vi "pp3_updateSideState.vi"(8 "error in (no error)":errorcluster, 9 "log queue in":refnum<queue>, 10 "Daq config In":T1={"Sound AO"="Dev6/ao0", "Shock intesity AO"="Dev6/ao1", "Code_LED DO"="Dev6/port1:2", "Switch DI"="Dev6/port1/line0", "Webcam"="cam9", "Sound AO task"="", "Sound card task"=0, "Shock intensity AO task"="", "Code_LED DO task"="", "Switch DI task"="", "AO <=> Sound card"=FALSE, "Sound card"=0, "sample rate"=100000.0, "Variable shock"=TRUE, "Webcam on"=FALSE, "Waveform memo"={"t0"=timestamp(0 s since 1904-01-01), "dt"=1.0, "Y"=[]}, "Tone trigger"="PFI1", "Master-9 DO"="", "Master-9 DO task"="Dev6/port0/line5:7"} {"sample rate" min=8000.0; "Sound card task" format="%.0x"}, 11 "State In":T4={"Curr  tr"=0, "Curr (ms)"=0, "Cum (ms)"=0, "Run loop diff"=0, "Tone countdown (ms)"=0, "Countdown (ms)"=0, "Curr State"=enum."0 NULL", "Prev State"=enum."1 Habituation", "Rw"=FALSE, "Sw"=FALSE, "Tone\nGate"=FALSE, "Punish"=FALSE, "Current DAQ DO Int"=0, "Current Loaded Trial"={"Trial Type Number"=1, "Trial Type"=enum."GO", "Trial Weight"=100, "Shock (mA)"=0.3, "Duration (ms)"=0.25, "Sound Type"=enum."04 FM Sweep", "Stim P1"=4000.0, "Stim P2"=0.0, "Stim P3"=0.0, "Stim P4"=2000.0, "DAQ Amplitude (V)"=0.25}, "Next Trial (for display purposes)"={"Trial Type Number"=1, "Trial Type"=enum."GO", "Trial Weight"=100, "Shock (mA)"=0.3, "Duration (ms)"=0.25, "Sound Type"=enum."04 FM Sweep", "Stim P1"=4000.0, "Stim P2"=0.0, "Stim P3"=0.0, "Stim P4"=2000.0, "DAQ Amplitude (V)"=0.25}, "Total trials memo"=0, "State start cum memo (ms)"=0, "Last dur jump time memo (ms)"=0, "Last dur shock time memo (ms)"=0, "Tone repeat memo (ms)"=0, "Webcam on"=FALSE, "Webcam recording"=FALSE, "State update flag"=FALSE, "Last loaded shock voltage"=0.0, "Vid upd"=enum."0"} {"Current DAQ DO Int" format="%016b"; "Next Trial (for display purposes)"."DAQ Amplitude (V)" min=0.0 max=5.0 format="%_4g"; "Next Trial (for display purposes)"."Shock (mA)" min=-1.0 max=5.0; "Next Trial (for display purposes)"."Trial Weight" step=1; "Next Trial (for display purposes)"."Duration (ms)" min=0.0 max=1.0; "Next Trial (for display purposes)"."Trial Type Number" min=1 max=256 step=1; "Current Loaded Trial"."DAQ Amplitude (V)" min=0.0 max=5.0 format="%_4g"; "Current Loaded Trial"."Shock (mA)" min=-1.0 max=5.0; "Current Loaded Trial"."Trial Weight" step=1; "Current Loaded Trial"."Duration (ms)" min=0.0 max=1.0; "Current Loaded Trial"."Trial Type Number" min=1 max=256 step=1}) -> (0 "error out":errorcluster, 1 "log queue out":refnum<queue>, 3 "State Out":T4={"Curr  tr"=0, "Curr (ms)"=0, "Cum (ms)"=0, "Run loop diff"=0, "Tone countdown (ms)"=0, "Countdown (ms)"=0, "Curr State"=enum."0 NULL", "Prev State"=enum."1 Habituation", "Rw"=FALSE, "Sw"=FALSE, "Tone\nGate"=FALSE, "Punish"=FALSE, "Current DAQ DO Int"=0, "Current Loaded Trial"={"Trial Type Number"=1, "Trial Type"=enum."GO", "Trial Weight"=100, "Shock (mA)"=0.3, "Duration (ms)"=0.25, "Sound Type"=enum."04 FM Sweep", "Stim P1"=4000.0, "Stim P2"=0.0, "Stim P3"=0.0, "Stim P4"=2000.0, "DAQ Amplitude (V)"=0.25}, "Next Trial (for display purposes)"={"Trial Type Number"=1, "Trial Type"=enum."GO", "Trial Weight"=100, "Shock (mA)"=0.3, "Duration (ms)"=0.25, "Sound Type"=enum."04 FM Sweep", "Stim P1"=4000.0, "Stim P2"=0.0, "Stim P3"=0.0, "Stim P4"=2000.0, "DAQ Amplitude (V)"=0.25}, "Total trials memo"=0, "State start cum memo (ms)"=0, "Last dur jump time memo (ms)"=0, "Last dur shock time memo (ms)"=0, "Tone repeat memo (ms)"=0, "Webcam on"=FALSE, "Webcam recording"=FALSE, "State update flag"=FALSE, "Last loaded shock voltage"=0.0, "Vid upd"=enum."0"} {"Current DAQ DO Int" format="%016b"; "Next Trial (for display purposes)"."DAQ Amplitude (V)" min=0.0 max=5.0 format="%_4g"; "Next Trial (for display purposes)"."Shock (mA)" min=-1.0 max=5.0; "Next Trial (for display purposes)"."Trial Weight" step=1; "Next Trial (for display purposes)"."Duration (ms)" min=0.0 max=1.0; "Next Trial (for display purposes)"."Trial Type Number" min=1 max=256 step=1; "Current Loaded Trial"."DAQ Amplitude (V)" min=0.0 max=5.0 format="%_4g"; "Current Loaded Trial"."Shock (mA)" min=-1.0 max=5.0; "Current Loaded Trial"."Trial Weight" step=1; "Current Loaded Trial"."Duration (ms)" min=0.0 max=1.0; "Current Loaded Trial"."Trial Type Number" min=1 max=256 step=1}, 4 "State timeout":bool, 5 "vid display":bool, 6 "Side change":bool)   [LabVIEW 2013]
uses:
  pp3_CTL_StateInfo.ctl
  pp3_CTL_State.ctl
  pp3_CTL_Trial.ctl
  pp3_CTL_TrialType.ctl
  labolabo2/waveforms/WFTypes.ctl
  CTL_pp3c_DaqStatus.ctl
  <vilib>/userdefined/High Color/IMAQdx.ctl
  <vilib>/sound2/lvsound2.llb/Sound Output Task ID.ctl
  <vilib>/DAQmx/read.llb/DAQmx Read (Digital Bool 1Line 1Point).vi
  <vilib>/DAQmx/miscellaneous.llb/DAQmx Fill In Error Info.vi
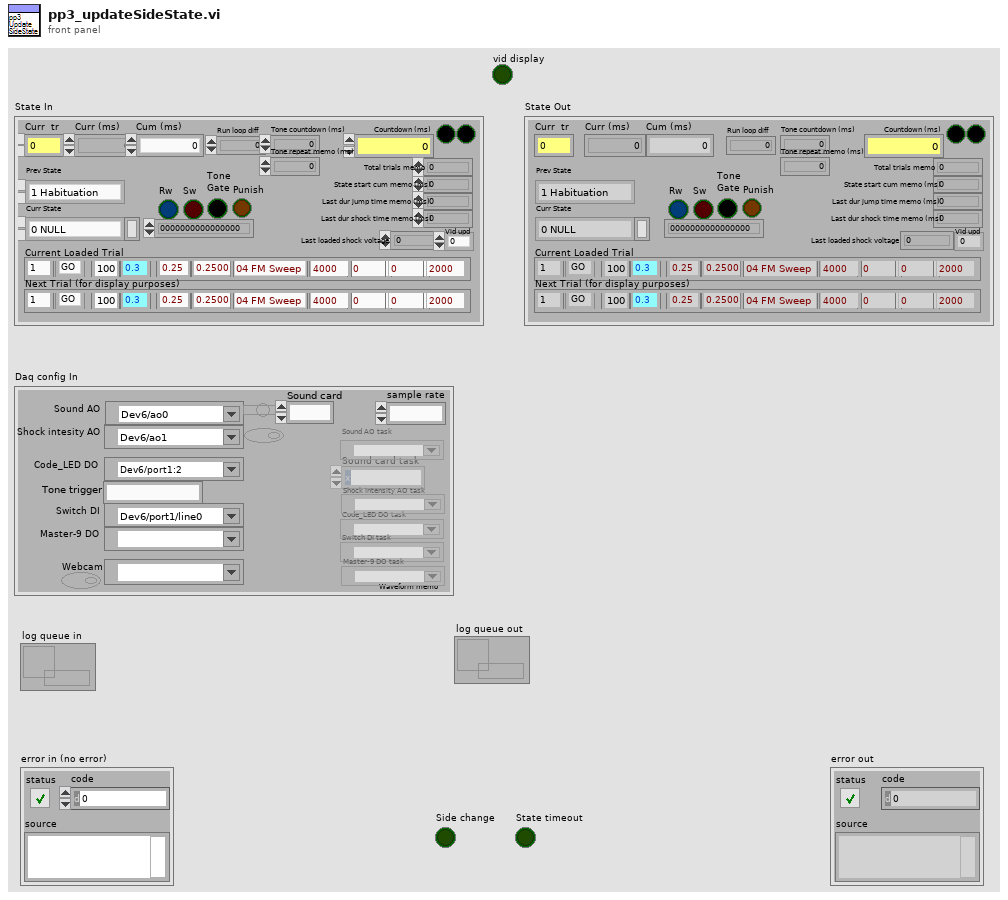
[diagram p1: front panel]
types:
  T1 = typedef "CTL_pp3c_DaqStatus.ctl" = cluster{"Sound AO":tag, "Shock intesity AO":tag, "Code_LED DO":tag, "Switch DI":tag, "Webcam":T2, "Sound AO task":refnum<k21>, "Sound card task":T3, "Shock intensity AO task":refnum<k21>, "Code_LED DO task":refnum<k21>, "Switch DI task":refnum<k21>, "AO <=> Sound card":bool, "Sound card":u32, "sample rate":dbl, "Variable shock":bool, "Webcam on":bool, "Waveform memo":waveform(dbl), "Tone trigger":string, "Master-9 DO":tag, "Master-9 DO task":refnum<k21>}
  T2 = typedef "IMAQdx.ctl" = refnum<k21>
  T3 = typedef "Sound Output Task ID.ctl" = u32
  T4 = typedef "pp3_CTL_StateInfo.ctl" = cluster{"Curr  tr":u16, "Curr (ms)":u32, "Cum (ms)":i64, "Run loop diff":i64, "Tone countdown (ms)":i64, "Countdown (ms)":i64, "Curr State":T5, "Prev State":T5, "Rw":bool, "Sw":bool, "Tone\nGate":bool, "Punish":bool, "Current DAQ DO Int":u16, "Current Loaded Trial":T6, "Next Trial (for display purposes)":T6, "Total trials memo":i64, "State start cum memo (ms)":i64, "Last dur jump time memo (ms)":i64, "Last dur shock time memo (ms)":i64, "Tone repeat memo (ms)":i64, "Webcam on":bool, "Webcam recording":bool, "State update flag":bool, "Last loaded shock voltage":dbl, "Vid upd":enum16{"0", "1", "2", "3", "4", "5", "6", "7", "8", "9"}}
  T5 = typedef "pp3_CTL_State.ctl" = enum8{"0 NULL", "1 Habituation", "2 (Load Trial)", "3 Stay Period", "4 Load Audio/Click Delay", "5 GO Trial", "6 GO Jumped", "7 GO Timeout", "8 NOGO Trial", "9 NOGO Jumped", "10 NOGO Timeout", "11 TEST Trial", "12 TEST Jumped", "13 TEST Timeout", "14 Intertrial Interval", "15 Done"}
  T6 = typedef "pp3_CTL_Trial.ctl" = cluster{"Trial Type Number":i16, "Trial Type":T7, "Trial Weight":u32, "Shock (mA)":dbl, "Duration (ms)":dbl, "Sound Type":T8, "Stim P1":dbl, "Stim P2":dbl, "Stim P3":dbl, "Stim P4":dbl, "DAQ Amplitude (V)":dbl}
  T7 = typedef "pp3_CTL_TrialType.ctl" = enum16{"OFF", "GO", "NOGO", "TEST"}
  T8 = typedef "WFTypes.ctl" = enum16{"00 NULL", "01 DC", "02 Noise", "03 Pure Tone", "04 FM Sweep"}
  T9 = enum16{"0", "1", "2", "3", "4", "5", "6", "7", "8", "9"}
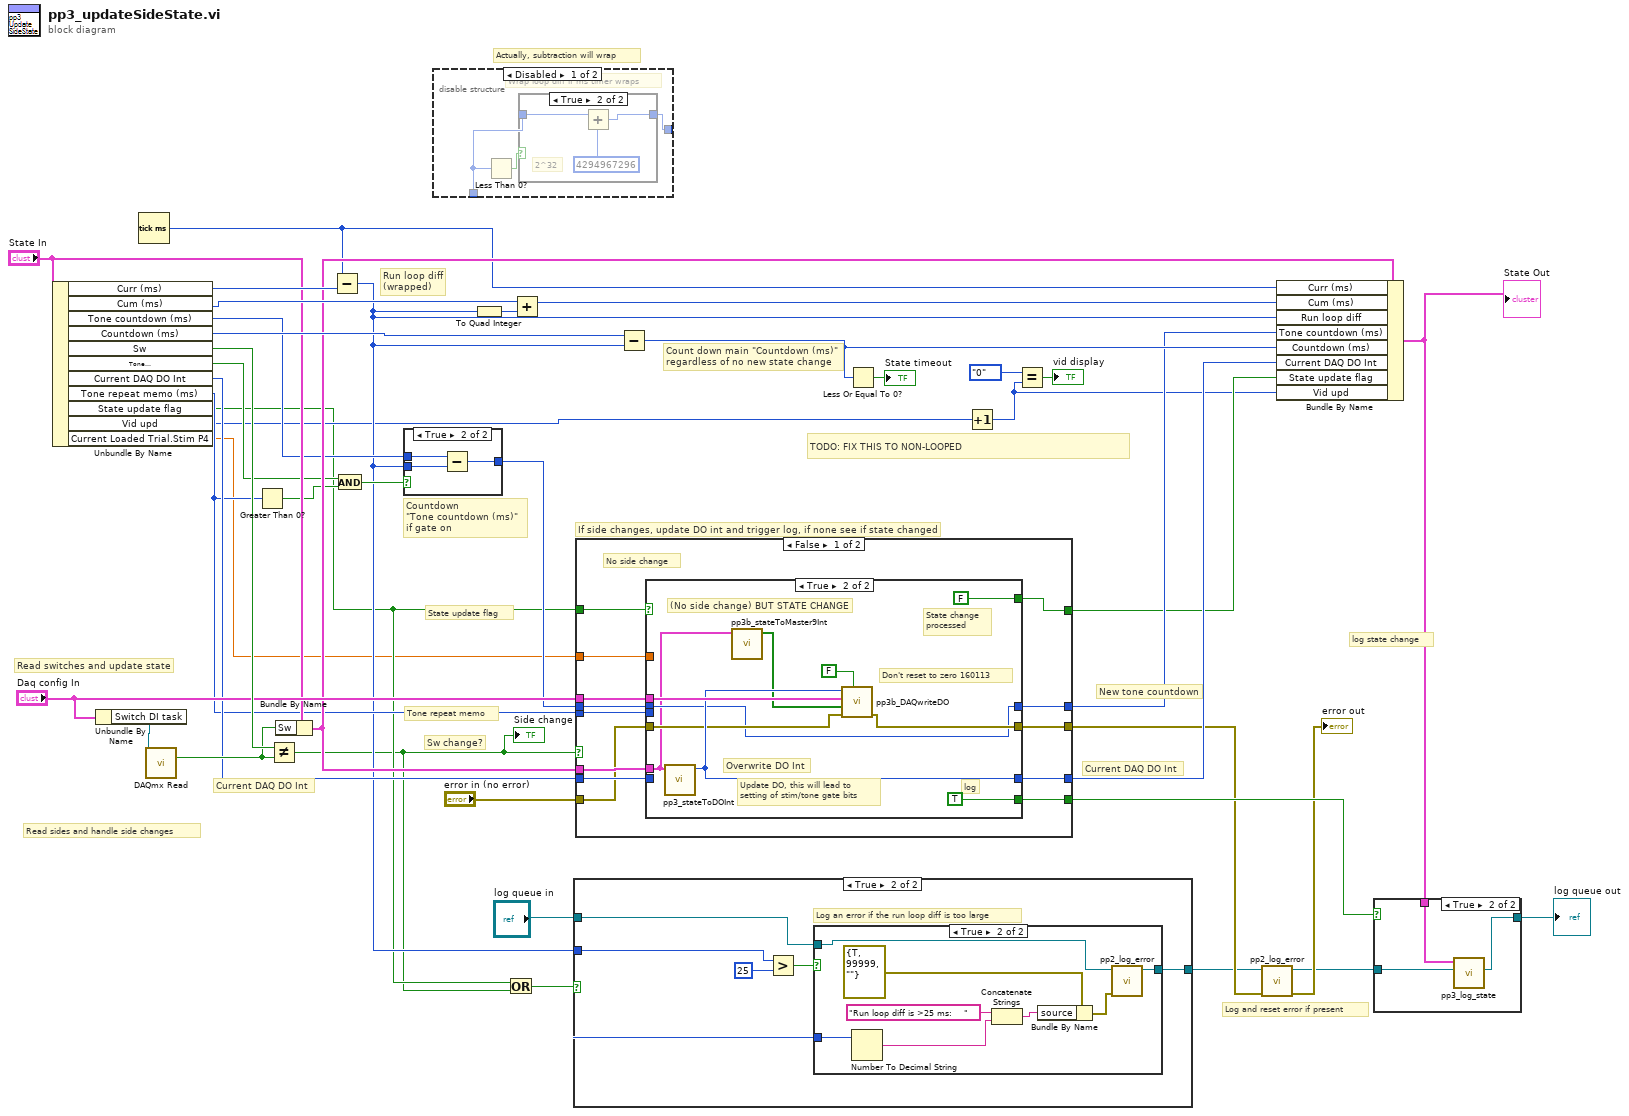
[diagram p0: block diagram]
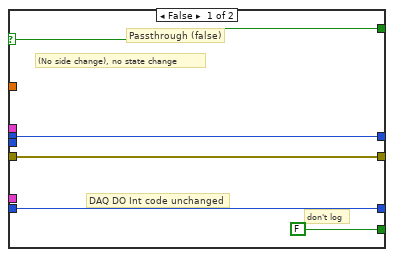
[diagram p8: hidden frame]
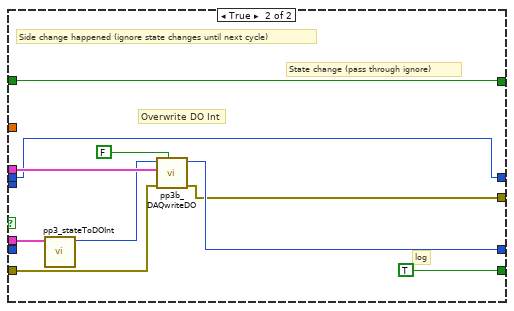
[diagram p9: hidden frame]
diagram:
  # "TODO: FIX THIS TO NON-LOOPED"
  # "Actually, subtraction will wrap"
  # "Log and reset error if present"
  # "New tone countdown"
  # "Countdown \n\"Tone countdown (ms)\" \nif gate on"
  # "Read switches and update state"
  # "Tone repeat memo"
  # "Sw change?"
  # "Current DAQ DO Int"
  # "Current DAQ DO Int"
  # "Count down main \"Countdown (ms)\" \nregardless of no new state change"
  # "State update flag"
  # "Run loop diff\n(wrapped)"
  # "If side changes, update DO int and trigger log, if none see if state changed"
  # "Read sides and handle side changes"
  # "log state change"
  n1 = Unbundle By Name("State In") -> ("Curr (ms)"=w42:u32, "Cum (ms)"=w41:i64, "Tone countdown (ms)"=w26:i64, "Countdown (ms)"=w39:i64, "Sw"=w37:bool, "Tone\nGate"=w16:bool, "Current DAQ DO Int"=w18:u16, "Tone repeat memo (ms)"=w14:i64, "State update flag"=w3:bool, "Vid upd"=w8:T9, "Current Loaded Trial.Stim P4"=w1:dbl)
  n2 = Unbundle By Name("Daq config In") -> ("Switch DI task"=w38:refnum<k21>)
  n3 = Tick Count (ms)() -> (millisecond timer value=w23:u32)
  n4 = call-poly <vilib>:"DAQmx Read.vi"("task/channels in"=w38) -> ("data"=w24:bool)  [unwired: 12 in, 2 out]
  n5 = Greater Than 0?(x=w14) -> (x > 0?=w15:bool)
  n6 = Not Equal?(x=w37, y=w24) -> (x != y?=w2:bool)
  "Side change" <- w2
  n7 = Bundle By Name(cluster="State In", "Sw"=w24) -> (w27:T4)
  n8 = Subtract(x=w23, y=w42) -> (x-y=w13:u32)
  n9 = And(x=w16, y=w15) -> (x .and. y?=w17:bool)
  n10 = case shown="True" w17 {
    tunnel: [w43 w44] -> w25
    tunnel: w26 -> [w43 w46]
    tunnel: w13 -> [_ w45]
    frame False {
      # "Passthrough if\ntone gate off"
    }
    frame True {
      n11 = Subtract(x=w46, y=w45) -> (x-y=w44:i64)
    }
  }
  n12 = disable-structure shown="Disabled" {
    disable-tunnel: [w48 _] -> _
    disable-tunnel: [w47 _] -> _
    frame Disabled {
      # "Wrap loop diff if ms timer wraps"
      n13 = Less Than 0?(x=w48) -> (x < 0?=w49:bool)
      n14 = case shown="True" w49 {
        tunnel: [w50 w52] -> w48
        tunnel: [w50 w53] -> w47
        frame False {
        }
        frame True {
          # "2^32"
          n15 = Add(x=w52, y=i64 4294967296) -> (x+y=w53:i64)
        }
      }
    }
    frame Enabled {
    }
  }
  n16 = To Quad Integer(1:w13) -> (0:w22:i64)
  n17 = Or(x=w3, y=w2) -> (x .or. y?=w4:bool)
  n18 = Add(x=w41, y=w22) -> (x+y=w40:i64)
  n19 = case shown="True" w4 {
    tunnel: w13 -> [_ w57]
    tunnel: "log queue in" -> [w54 w56]
    tunnel: [w54 w55] -> w11
    frame False {
    }
    frame True {
      # "Log an error if the run loop diff is too large"
      n20 = Greater?(x=w57, y=u32 25) -> (0:w58:bool)
      n21 = case shown="True" w58 {
        tunnel: w57 -> [_ w67]
        tunnel: w56 -> [w60 w62]
        tunnel: [w60 w61] -> w55
        frame False {
        }
        frame True {
          n22 = Number To Decimal String(number=w67) -> (decimal integer string=w64:string)  [unwired: 1 in]
          n23 = Concatenate Strings("Run loop diff is >25 ms:    " ("string"), w64) -> (w66:string)
          n24 = Bundle By Name(cluster=errorcluster {"status"=TRUE, "code"=99999, "source"=""} ("error in (no error)"), "source"=w66) -> (w63:errorcluster)
          n25 = call "pp2_log_error.vi"("error in (no error)"=w63, "queue in"=w62) -> ("queue out"=w61:refnum<queue>)  [unwired: 6 in, 1 out]
        }
      }
    }
  }
  n26 = case shown="False" w2 {
    tunnel: "Daq config In" -> [w75 w104]
    tunnel: [w80 w103] -> w28
    tunnel: w18 -> [w81 _]
    tunnel: "error in (no error)" -> [w74 w102]
    tunnel: [w78 w101] -> w20
    tunnel: [w79 TRUE] -> w32
    tunnel: w14 -> [w73 _]
    tunnel: w3 -> [w77 w98]
    tunnel: w27 -> [w76 w100]
    tunnel: [w72 w99] -> w30
    tunnel: w25 -> [w71 w99]
    tunnel: [w70 w98] -> w21
    tunnel: w1 -> [w69 _]
    frame False {
      # "No side change"
      n27 = case shown="True" w77 {
        selector: w77 -> [w83 _]
        tunnel: w81 -> [w82 _]
        tunnel: [w82 w95] -> w80
        tunnel: w75 -> [_ w96]
        tunnel: [FALSE TRUE] -> w79
        tunnel: w74 -> [w84 w93]
        tunnel: [w84 w92] -> w78
        tunnel: w76 -> [_ w88]
        tunnel: w71 -> [w85 w91]
        tunnel: w73 -> [_ _]
        tunnel: [w85 w91] -> w72
        tunnel: [w83 FALSE] -> w70
        tunnel: w69 -> [_ _]
        frame False {
          # "Passthrough (false)"
          # "don't log"
          # "DAQ DO Int code unchanged"
          # "(No side change), no state change"
        }
        frame True {
          # "Don't reset to zero 160113"
          # "State change\nprocessed"
          # "log"
          # "Overwrite DO Int"
          # "Update DO, this will lead to\nsetting of stim/tone gate bits"
          # "(No side change) BUT STATE CHANGE"
          n28 = call "pp3_stateToDOInt.vi"("State In"=w88) -> ("DAQ Output Int"=w95:u16)  [unwired: 10 in]
          n29 = call "pp3b_stateToMaster9Int.vi"("State In"=w88) -> ("Master-9 Output Array"=w87:bool[])  [unwired: 10 in]
          n30 = call "pp3b_DAQwriteDO.vi"("Reset to zero"=FALSE, "error in (no error)"=w93, "Master-9 Digital"=w87, "Daq config"=w96, "DAQ Digital In"=w95) -> ("error out"=w92:errorcluster)  [unwired: 6 in]
        }
      }
    }
    frame True {
      # "State change (pass through ignore)"
      # "log"
      # "Side change happened (ignore state changes until next cycle)"
      # "Overwrite DO Int"
      n31 = call "pp3_stateToDOInt.vi"("State In"=w100) -> ("DAQ Output Int"=w103:u16)  [unwired: 10 in]
      n32 = call "pp3b_DAQwriteDO.vi"("Reset to zero"=FALSE, "error in (no error)"=w102, "Daq config"=w104, "DAQ Digital In"=w103) -> ("error out"=w101:errorcluster)  [unwired: 7 in]
    }
  }
  n33 = Subtract(x=w39, y=w13) -> (x-y=w36:i64)
  n34 = Less Or Equal To 0?(x=w36) -> (x <= 0?=→"State timeout":bool)
  n35 = Increment(x=w8) -> (x+1=w7:T9)
  n36 = Equal?(x=T9."0", y=w7) -> (x = y?=→"vid display":bool)
  n37 = call "pp2_log_error.vi"("error in (no error)"=w20, "queue in"=w11) -> ("error out"=→"error out":errorcluster, "queue out"=w10:refnum<queue>)  [unwired: 6 in]
  n38 = Bundle By Name(cluster=w27, "Curr (ms)"=w23, "Cum (ms)"=w40, "Run loop diff"=w13, "Tone countdown (ms)"=w30, "Countdown (ms)"=w36, "Current DAQ DO Int"=w28, "State update flag"=w21, "Vid upd"=w7) -> (w31:T4)
  "State Out" <- w31
  n39 = case shown="True" w32 {
    tunnel: w31 -> [_ w109]
    tunnel: w10 -> [w106 w108]
    tunnel: [w106 w107] -> w9
    frame False {
    }
    frame True {
      n40 = call "pp3_log_state.vi"("queue in"=w108, "State In"=w109) -> ("queue out"=w107:refnum<queue>)  [unwired: 9 in]
    }
  }
  "log queue out" <- w9
